vi "N9030B_DG5252_0916.vi"() -> ()   [LabVIEW 2017]
uses:
  <vilib>/picture/cartesn2.llb/XY Plot Type.ctl
  <vilib>/Utility/file.llb/Write Delimited Spreadsheet (DBL).vi
  <vilib>/Utility/file.llb/Write Delimited Spreadsheet (string).vi
  <instrlib>/Keysight XSAn/Keysight XSAn.lvlib
panel:
  in  "XY Plot Cosmetics":T2(array[cluster])=[{"Color Box"=3381759, "plot type"=enum."connected squares", "baseline"=0.0}, {"Color Box"=6618880, "plot type"=enum."connected points", "baseline"=0.0}, {"Color Box"=16768018, "plot type"=enum."connected circles", "baseline"=0.0}]
  out "?":picture
  in  "csv header":string[](array[string])
  in  "folder name":string
  out "element":dbl
  out "sweep":bool
  in  "stop":bool
  in  "Path":path=path "d:/"
  out "actual points":i32
  in  "Array":cluster{"Numeric":dbl, "Numeric 2":dbl}[](array[cluster])
  in  "frequency points":T3 {"point 2 (Hz)" format="%#_6p"; "point 1 (Hz)" format="%#_6p"; "frequency 1 (Hz)" format="%#_6p"}
  in  "Keysight N9030B":refnum<visa-resource-name> caption="resource name"
  in  "Rigol DG5252":refnum<visa-resource-name>
  in  "Rigol DG5252":T4={"start frequency (MHz)"=150.0, "frequency spacing (MHz)"=1.0, "stop frequency (MHz)"=250.0, "sweep frequency"=FALSE}
  out "error out":errorcluster {"code" format="%.0x"}
  in  "Keysight N9030B":T5={"center frequency"=15000.0, "span"=5000.0, "noise floor (dBm)"=0.0} {"span" format="%#_6p"; "center frequency" format="%#_6p"}
  out "amplitude":dbl[](array[numeric])
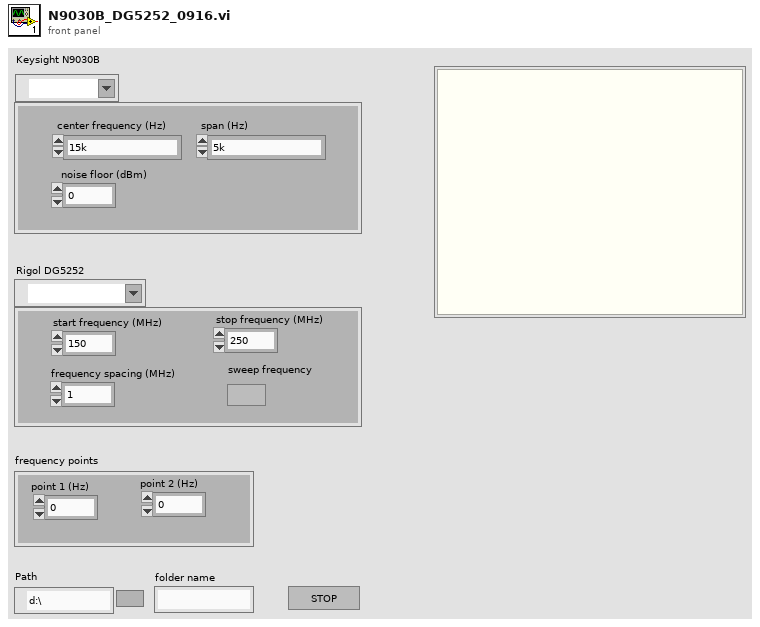
[diagram p1: front panel]
types:
  T1 = typedef "XY Plot Type.ctl" = enum16{"points", "squares", "circles", "connected points", "connected squares", "connected circles", "comb plot", "sized scatter plot", "sized-colored scatter plot", "min-max lines"}
  T2 = cluster{"Color Box":u32, "plot type":T1, "baseline":dbl}[]
  T3 = cluster{"frequency 1 (Hz)":dbl, "point 1 (Hz)":dbl, "point 2 (Hz)":dbl}
  T4 = cluster{"start frequency (MHz)":dbl, "frequency spacing (MHz)":dbl, "stop frequency (MHz)":dbl, "sweep frequency":bool}
  T5 = cluster{"center frequency":dbl, "span":dbl, "noise floor (dBm)":dbl}
  T6 = cluster{"Array":cluster{"Numeric":dbl, "Numeric 2":dbl}[]}
  T7 = cluster{"Array":cluster{"Numeric":dbl, "Numeric 2":dbl}[]}[]
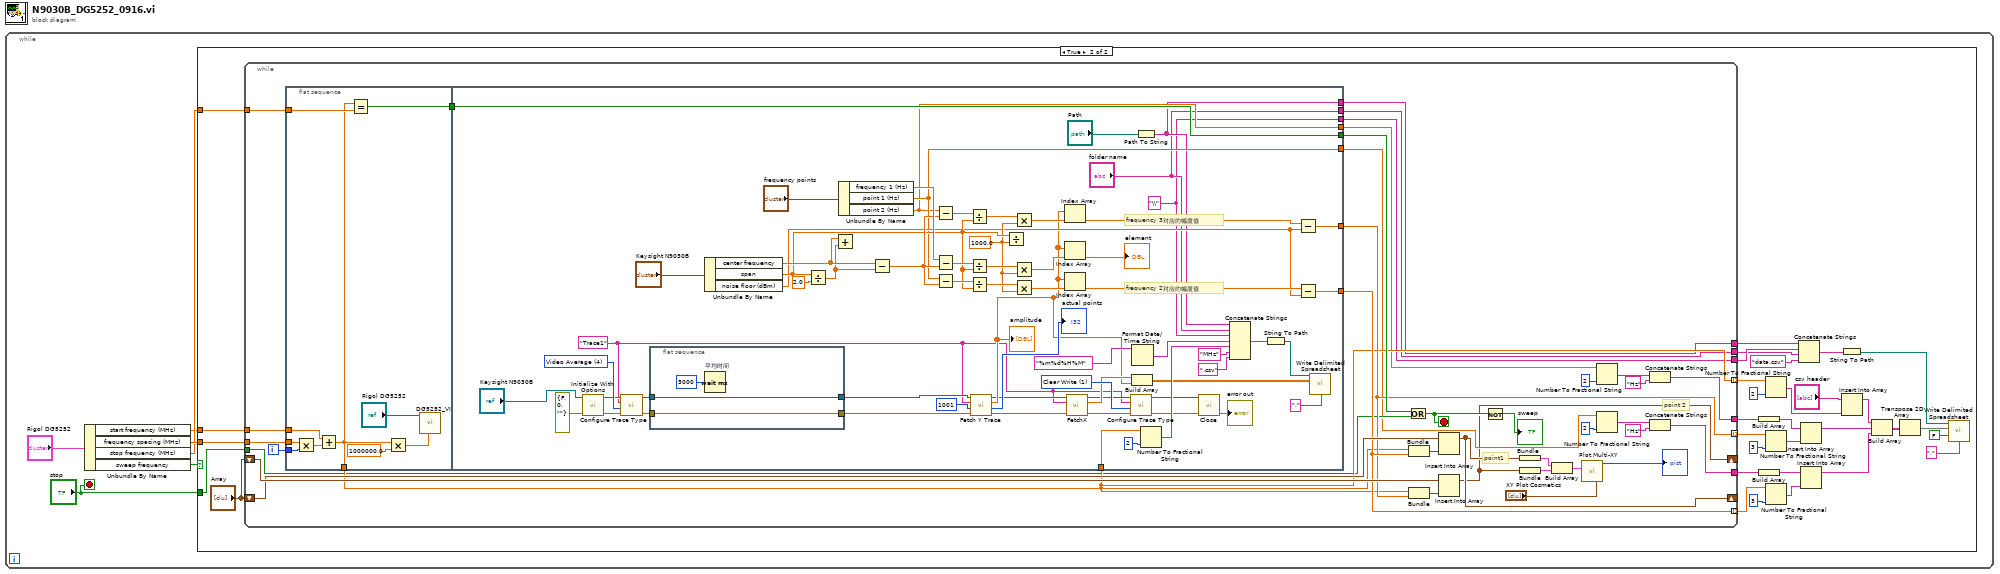
[diagram p0: block diagram]
diagram:
  n1 = while {
    stop <- "stop" stop-if-true
    n2 = Unbundle By Name("Rigol DG5252") -> ("start frequency (MHz)"=w2:dbl, "frequency spacing (MHz)"=w4:dbl, "stop frequency (MHz)"=w3:dbl, "sweep frequency"=w5:bool)
    n3 = case shown="True" w5 {
      tunnel: w2 -> [_ w36]
      tunnel: w4 -> [_ w38]
      tunnel: w3 -> [_ w35]
      tunnel: "stop" -> [_ w33]
      frame False {
      }
      frame True {
        n4 = while {
          tunnel: w36 -> [w74]
          tunnel: w38 -> [w73]
          tunnel: w35 -> [w71]
          shift-right: [w47] -> _
          shift-left: "Array" -> [w69]
          shift-right: [w48] -> _
          shift-left: "Array" -> [w68]
          tunnel: [w62] -> w27 mode=indexing
          tunnel: [w61] -> w16 mode=indexing
          tunnel: [w60] -> w22 mode=indexing
          tunnel: w33 -> [w59]
          tunnel: [w54] -> w29
          tunnel: [w49] -> w18
          tunnel: [w41] -> w12
          tunnel: [w40] -> w11
          tunnel: [w39] -> w10
          i -> [w72]
          stop <- w64 stop-if-true
          # "point 2"
          # "point1"
          n5 = flat-sequence {
            tunnel: w74 -> [w83]
            tunnel: w73 -> [w82]
            tunnel: w72 -> [w81]
            tunnel: w71 -> [w77]
            tunnel: [w76] -> w70
            tunnel: [w75] -> w60
            tunnel: [w148] -> w65
            tunnel: w70 -> [w148]
            tunnel: [w113] -> w62
            tunnel: [w116] -> w61
            tunnel: w60 -> [w127]
            tunnel: [w110] -> w58
            tunnel: [w109] -> w53
            tunnel: [w87] -> w41
            tunnel: ["folder name"] -> w40
            tunnel: [w85] -> w39
            frame #0 {
              n6 = Multiply(x=w82, y=w81) -> (x*y=w80:dbl)
              n7 = Add(x=w83, y=w80) -> (x+y=w75:dbl)
              n8 = Equal?(x=w75, y=w77) -> (x = y?=w76:bool)
              n9 = Multiply(x=w75, y=1000000.0) -> (x*y=w78:dbl)
              n10 = call "DG5252_VI.vi"("Frequency (1000 Hz)"=w78, "VISA resource name"="Rigol DG5252") -> ()  [unwired: 10 in]
            }
            frame #1 {
              w103 = 1 items=["Clear Write"=1, "Maximum Hold"=2, "Minimum Hold"=3, "Video Average"=4, "View"=5, "Store"=6] ("trace type (Clear Write)")
              w108 = 4 items=["Clear Write"=1, "Maximum Hold"=2, "Minimum Hold"=3, "Video Average"=4, "View"=5, "Store"=6] ("trace type (Clear Write)")
              w88 = "Trace1" ("trace name")
              w85 = "\\" ("string")
              w120 = 1000.0 ("y")
              # "frequency 3对应的幅度值"
              # "frequency 2对应的幅度值"
              n11 = call <instrlib>:"Initialize With Options.vi"("error in (no error)"=errorcluster {"status"=FALSE, "code"=0, "source"=""}, "resource string"="Keysight N9030B") -> ("error out"=w106:errorcluster, "instrument handle out"=w107:refnum<k15>)  [unwired: 8 in]
              n12 = call <instrlib>:"Configure Trace Type.vi"("error in (no error)"=w106, "trace type (Clear Write)"=w108, "trace name"=w88, "instrument handle"=w107) -> ("error out"=w104:errorcluster, "instrument handle out"=w105:refnum<k15>)  [unwired: 6 in]
              n13 = flat-sequence {
                tunnel: [w149] -> w139
                tunnel: [w150] -> w140
                tunnel: w105 -> [w150]
                tunnel: w104 -> [w149]
                frame #0 {
                  n14 = Wait (ms) "平均时间"(milliseconds to wait=u32 3000) -> ()  [unwired: 1 out]
                }
              }
              n15 = Unbundle By Name("Keysight N9030B") -> ("center frequency"=w137:dbl, "span"=w122:dbl, "noise floor (dBm)"=w114:dbl)
              n16 = Divide(x=w122, y=2.0) -> (x/y=w136:dbl)
              n17 = Add(x=w137, y=w136) -> ()  [unwired: 1 out]
              n18 = Unbundle By Name("frequency points") -> ("frequency 1 (Hz)"=w125:dbl, "point 1 (Hz)"=w110:dbl, "point 2 (Hz)"=w109:dbl)
              n19 = Subtract(x=w137, y=w136) -> (x-y=w124:dbl)
              n20 = Subtract(x=w109, y=w124) -> (x-y=w132:dbl)
              n21 = Subtract(x=w125, y=w124) -> (x-y=w123:dbl)
              n22 = Subtract(x=w110, y=w124) -> (x-y=w135:dbl)
              n23 = Divide(x=w132, y=w122) -> (x/y=w131:dbl)
              n24 = Divide(x=w123, y=w122) -> (x/y=w121:dbl)
              n25 = Divide(x=w135, y=w122) -> (x/y=w134:dbl)
              n26 = call <instrlib>:"Fetch Y Trace.vi"("error in (no error)"=w139, "array length"=1001, "trace name"=w88, "instrument handle"=w140) -> ("error out"=w93:errorcluster, "actual points"=→"actual points":i32, "amplitude"=w99:dbl[], "instrument handle out"=w94:refnum<k15>)  [unwired: 4 in]
              "amplitude" <- w99
              n27 = Divide(x=w122, y=w120) -> ()  [unwired: 1 out]
              n28 = Multiply(x=w131, y=w120) -> (x*y=w130:dbl)
              n29 = Multiply(x=w121, y=w120) -> (x*y=w119:dbl)
              n30 = Multiply(x=w134, y=w120) -> (x*y=w133:dbl)
              n31 = Index Array(array=w99, index=w130) -> (element=w117:dbl)
              n32 = Index Array(array=w99, index=w119) -> (element=→"element":dbl)
              n33 = Index Array(array=w99, index=w133) -> (element=w115:dbl)
              n34 = call <instrlib>:"FetchX.vi"("error in (no error)"=w93, "Trace"=w88, "instrument handle"=w94) -> ("error out"=w91:errorcluster, "Val"=w100:dbl[], "instrument handle out"=w92:refnum<k15>)  [unwired: 5 in, 1 out]
              n35 = call <instrlib>:"Configure Trace Type.vi"("error in (no error)"=w91, "trace type (Clear Write)"=w103, "trace name"=w88, "instrument handle"=w92) -> ("error out"=w101:errorcluster, "instrument handle out"=w102:refnum<k15>)  [unwired: 6 in]
              n36 = Build Array(w100, w99) -> (w98:dbl[][])
              n37 = Format Date/Time String(time format string (%c)="%m%d%H%M") -> (date/time string=w111:string)  [unwired: 2 in]
              n38 = Path To String(path="Path") -> (string=w87:string)
              n39 = Number To Fractional String(number=w127, precision (6)=i16 2) -> (F-format string=w112:string)  [unwired: 2 in]
              n40 = call <instrlib>:"Close.vi"("error in (no error)"=w101, "instrument handle"=w102) -> ("error out"=→"error out":errorcluster)  [unwired: 9 in]
              n41 = Concatenate Strings(w87, "folder name", w85, w111, w112, "MHz" ("string"), ".csv" ("string")) -> (w96:string)
              n42 = String To Path(string=w96) -> (path=w95:path)
              n43 = Subtract(x=w117, y=w114) -> (x-y=w116:dbl)
              n44 = Subtract(x=w115, y=w114) -> (x-y=w113:dbl)
              n45 = call-poly <vilib>:"Write Delimited Spreadsheet.vi"("file path (dialog if empty)"=w95, "2D data"=w98, "delimiter (\\t)"="," ("delimiter (\\t)")) -> ()  [unwired: 11 in, 2 out]
            }
          }
          n46 = Or(x=w65, y=w59) -> (x .or. y?=w64:bool)
          n47 = Bundle(w60, w62) -> (w67:cluster{dbl, dbl})  [unwired: 1 in]
          n48 = Bundle(w60, w61) -> (w66:cluster{dbl, dbl})  [unwired: 1 in]
          n49 = Insert Into Array(array=w68, new element=w67) -> (w48:cluster{"Numeric":dbl, "Numeric 2":dbl}[])  [unwired: 1 in]
          n50 = Insert Into Array(array=w69, new element=w66) -> (w47:cluster{"Numeric":dbl, "Numeric 2":dbl}[])  [unwired: 1 in]
          n51 = Not(x=w64) -> (.not. x?=→"sweep":bool)
          n52 = Bundle("Array"=w48) -> (w46:T6)  [unwired: 1 in]
          n53 = Bundle("Array"=w47) -> (w45:T6)  [unwired: 1 in]
          n54 = Build Array(w46, w45) -> (w44:T7)
          n55 = call <vilib>:"Plot Multi-XY.vi"("data"=w44, "XY plot cosmetics"="XY Plot Cosmetics") -> ("new picture"=→"?":picture)  [unwired: 13 in]
          n56 = Number To Fractional String(number=w53, precision (6)=i16 2) -> (F-format string=w51:string)  [unwired: 2 in]
          n57 = Number To Fractional String(number=w58, precision (6)=i16 2) -> (F-format string=w56:string)  [unwired: 2 in]
          n58 = Concatenate Strings(w51, "Hz" ("string")) -> (w49:string)
          n59 = Concatenate Strings(w56, "Hz" ("string")) -> (w54:string)
        }
        n60 = Build Array(w18) -> (w17:string[])
        n61 = Build Array(w29) -> (w28:string[])
        n62 = Number To Fractional String(number=w22, precision (6)=i16 2) -> (F-format string=w20:string[])  [unwired: 2 in]
        n63 = Number To Fractional String(number=w16, precision (6)=i16 3) -> (F-format string=w14:string[])  [unwired: 2 in]
        n64 = Number To Fractional String(number=w27, precision (6)=i16 3) -> (F-format string=w25:string[])  [unwired: 2 in]
        n65 = Concatenate Strings(w12, w11, w10, "data.csv" ("string")) -> (w8:string)
        n66 = Insert Into Array(array=w17, new element=w14) -> (w13:string[])  [unwired: 1 in]
        n67 = Insert Into Array(array=w28, new element=w25) -> (w24:string[])  [unwired: 1 in]
        n68 = String To Path(string=w8) -> (path=w7:path)
        n69 = Insert Into Array(array="csv header", new element=w20) -> (w19:string[])  [unwired: 1 in]
        n70 = Build Array(w19, w13, w24) -> (w32:string[][])
        n71 = Transpose 2D Array(2D array=w32) -> (transposed array=w31:string[][])
        n72 = call-poly <vilib>:"Write Delimited Spreadsheet.vi"("file path (dialog if empty)"=w7, "2D data"=w31, "append to file? (new file:F)"=FALSE, "delimiter (\\t)"="," ("delimiter (\\t)")) -> ()  [unwired: 10 in, 2 out]
      }
    }
  }
